vi "BME_Set_G05.vi"(0 "BME_G05P1 Settings":T2={"GateAB?"=FALSE, "Signal Type"=1, "InputTerminated?"=TRUE, "ClockEnabled?"=TRUE, "InternalClockPeriode(µs)"=1000000.0, "TriggerLevel"=1.25, "PresetValue"=0, "DivideBy"=8, "Clock Source"=1, "Gate Divider"=1, "PositiveGate?"=FALSE, "InternalTrigger?"=FALSE, "InternalArm?"=FALSE, "SWTrigger?"=FALSE, "RisingEdge?"=TRUE, "StopOnPreset?"=FALSE, "ResetWhenDone?"=FALSE, "TriggerEnabled?"=TRUE} {"Gate Divider" min=1 max=1000000; "Clock Source" items=["Internal Oscillator"=1, "External Trigger"=2, "Trigger & Oscillator"=3]; "Signal Type" items=["TTL"=1, "ECL"=2, "NIM"=3]}, 1 "DG_Number":i32, 5 "Chnl T":T1={" Delay (µs)"=0.0, "TriggerModulo"=1, "On? (false)"=FALSE, "PositiveVoltage?(true)"=TRUE, "50OhmTerminated? "=FALSE, "25OhmOutput?"=FALSE} {"TriggerModulo" min=1 max=1000000; "Delay (µs)" min=0.0 max=100000000.0 format="%.5f"}, 7 "Chnl A":T1={" Delay (µs)"=0.0, "TriggerModulo"=1, "On? (false)"=FALSE, "PositiveVoltage?(true)"=TRUE, "50OhmTerminated? "=FALSE, "25OhmOutput?"=FALSE} {"TriggerModulo" min=1 max=1000000; "Delay (µs)" min=0.0 max=100000000.0 format="%.5f"}, 9 "Chnl B":T1={" Delay (µs)"=0.0, "TriggerModulo"=1, "On? (false)"=FALSE, "PositiveVoltage?(true)"=TRUE, "50OhmTerminated? "=FALSE, "25OhmOutput?"=FALSE} {"TriggerModulo" min=1 max=1000000; "Delay (µs)" min=0.0 max=100000000.0 format="%.5f"}, 11 "error in (no error)":errorcluster) -> (8 "return value":i32, 15 "error out":errorcluster)   [LabVIEW 2009]
uses:
  BME_G05P1Settings.ctl
  SignalType.ctl
  ChnlWithModulo.ctl
  BME Beispiele/BME DLL/DelayGenerator.dll
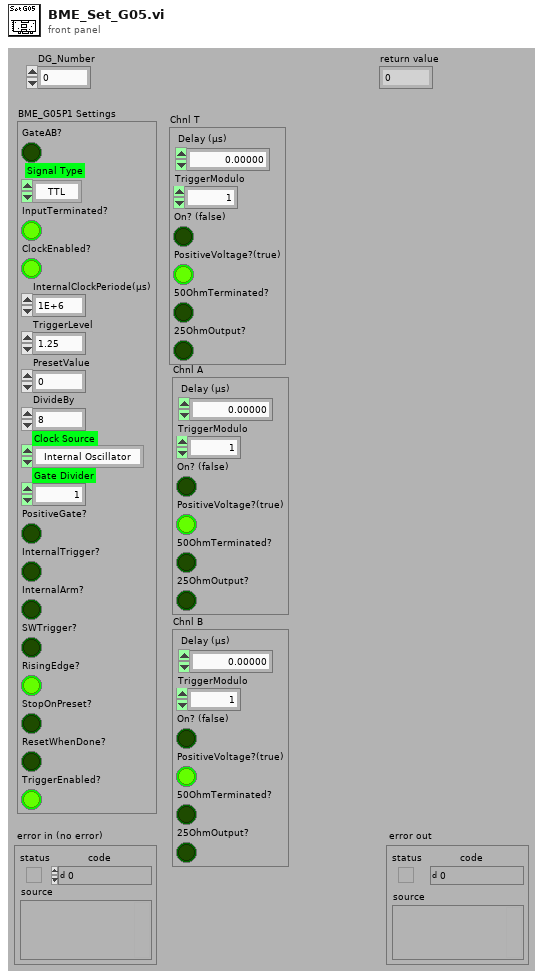
[diagram p1: front panel]
types:
  T1 = typedef "ChnlWithModulo.ctl" = cluster{" Delay (µs)":dbl, "TriggerModulo":u32, "On? (false)":bool, "PositiveVoltage?(true)":bool, "50OhmTerminated? ":bool, "25OhmOutput?":bool}
  T2 = typedef "BME_G05P1Settings.ctl" = cluster{"GateAB?":bool, "Signal Type":T3, "InputTerminated?":bool, "ClockEnabled?":bool, "InternalClockPeriode(µs)":dbl, "TriggerLevel":dbl, "PresetValue":i32, "DivideBy":i32, "Clock Source":u32, "Gate Divider":i32, "PositiveGate?":bool, "InternalTrigger?":bool, "InternalArm?":bool, "SWTrigger?":bool, "RisingEdge?":bool, "StopOnPreset?":bool, "ResetWhenDone?":bool, "TriggerEnabled?":bool}
  T3 = typedef "SignalType.ctl" = u32
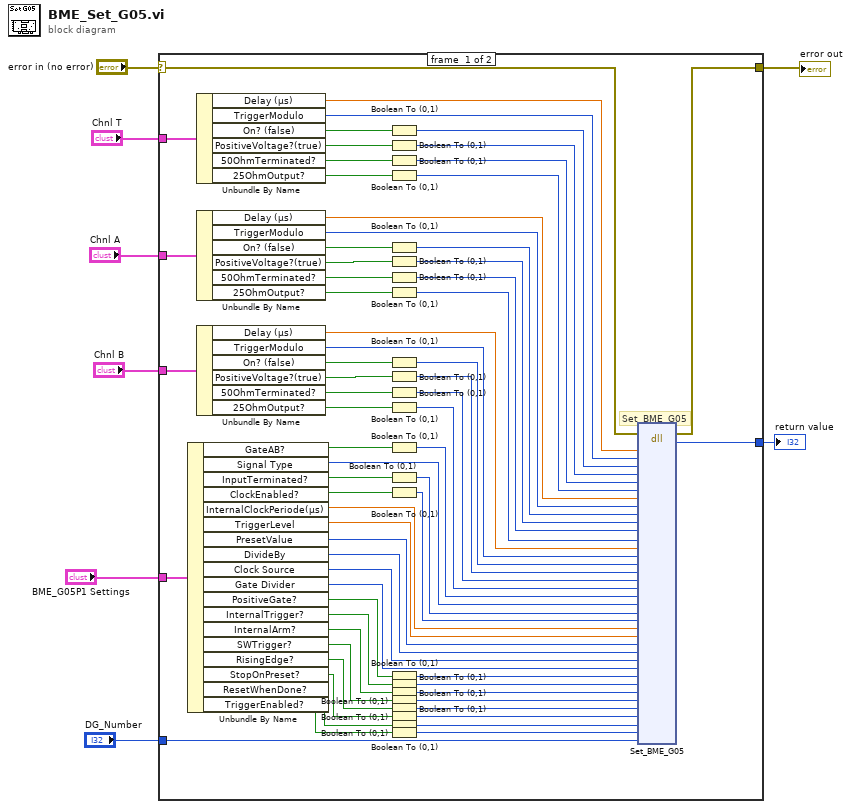
[diagram p0: block diagram]
diagram:
  n1 = case shown="No Error" "error in (no error)" {
    selector: "error in (no error)" -> [w9 w76]
    tunnel: "BME_G05P1 Settings" -> [w57 _]
    tunnel: "Chnl B" -> [w50 _]
    tunnel: "Chnl A" -> [w43 _]
    tunnel: "Chnl T" -> [w36 _]
    tunnel: [w34 _] -> w4
    tunnel: "DG_Number" -> [w33 _]
    tunnel: [w10 w76] -> w2
    frame #0 {
      # "Set_BME_G05"
      n2 = Unbundle By Name(w57) -> ("GateAB?"=w58:bool, "Signal Type"=w59:T3, "InputTerminated?"=w60:bool, "ClockEnabled?"=w61:bool, "InternalClockPeriode(µs)"=w62:dbl, "TriggerLevel"=w63:dbl, "PresetValue"=w64:i32, "DivideBy"=w65:i32, "Clock Source"=w66:u32, "Gate Divider"=w67:i32, "PositiveGate?"=w68:bool, "InternalTrigger?"=w69:bool, "InternalArm?"=w70:bool, "SWTrigger?"=w71:bool, "RisingEdge?"=w72:bool, "StopOnPreset?"=w73:bool, "ResetWhenDone?"=w74:bool, "TriggerEnabled?"=w75:bool)
      n3 = Unbundle By Name(w36) -> ("Delay (µs)"=w37:dbl, "TriggerModulo"=w38:u32, "On? (false)"=w39:bool, "PositiveVoltage?(true)"=w40:bool, "50OhmTerminated?"=w41:bool, "25OhmOutput?"=w42:bool)
      n4 = Unbundle By Name(w43) -> ("Delay (µs)"=w44:dbl, "TriggerModulo"=w45:u32, "On? (false)"=w46:bool, "PositiveVoltage?(true)"=w47:bool, "50OhmTerminated?"=w48:bool, "25OhmOutput?"=w49:bool)
      n5 = Unbundle By Name(w50) -> ("Delay (µs)"=w51:dbl, "TriggerModulo"=w52:u32, "On? (false)"=w53:bool, "PositiveVoltage?(true)"=w54:bool, "50OhmTerminated?"=w55:bool, "25OhmOutput?"=w56:bool)
      n6 = Boolean To (0,1)(Boolean=w39) -> (0, 1=w32:i16)
      n7 = Boolean To (0,1)(Boolean=w40) -> (0, 1=w31:i16)
      n8 = Boolean To (0,1)(Boolean=w41) -> (0, 1=w30:i16)
      n9 = Boolean To (0,1)(Boolean=w42) -> (0, 1=w29:i16)
      n10 = Boolean To (0,1)(Boolean=w46) -> (0, 1=w28:i16)
      n11 = Boolean To (0,1)(Boolean=w47) -> (0, 1=w27:i16)
      n12 = Boolean To (0,1)(Boolean=w48) -> (0, 1=w26:i16)
      n13 = Boolean To (0,1)(Boolean=w49) -> (0, 1=w25:i16)
      n14 = Boolean To (0,1)(Boolean=w53) -> (0, 1=w24:i16)
      n15 = Boolean To (0,1)(Boolean=w54) -> (0, 1=w23:i16)
      n16 = Boolean To (0,1)(Boolean=w55) -> (0, 1=w22:i16)
      n17 = Boolean To (0,1)(Boolean=w56) -> (0, 1=w21:i16)
      n18 = Boolean To (0,1)(Boolean=w58) -> (0, 1=w20:i16)
      n19 = Boolean To (0,1)(Boolean=w60) -> (0, 1=w19:i16)
      n20 = Boolean To (0,1)(Boolean=w61) -> (0, 1=w35:i16)
      n21 = Boolean To (0,1)(Boolean=w68) -> (0, 1=w18:i16)
      n22 = Boolean To (0,1)(Boolean=w69) -> (0, 1=w17:i16)
      n23 = Boolean To (0,1)(Boolean=w70) -> (0, 1=w16:i16)
      n24 = Boolean To (0,1)(Boolean=w71) -> (0, 1=w15:i16)
      n25 = Boolean To (0,1)(Boolean=w72) -> (0, 1=w14:i16)
      n26 = Boolean To (0,1)(Boolean=w73) -> (0, 1=w13:i16)
      n27 = Boolean To (0,1)(Boolean=w74) -> (0, 1=w12:i16)
      n28 = Boolean To (0,1)(Boolean=w75) -> (0, 1=w11:i16)
      n29 = dll-call lib="C:/Dokumente und Einstellungen/A2.5/Desktop/BME Beispiele/BME DLL/DelayGenerator.dll" fn="Set_BME_G05"(error in=w9, "T_0"=w37, "T0_output_modulo"=w38, "T0_active"=w32, "T0_pos"=w31, "T0_term"=w30, "T0_hdr"=w29, "T_a"=w44, "Ta_output_modulo"=w45, "A_active"=w28, "A_pos"=w27, "A_term"=w26, "A_hdr"=w25, "T_b"=w51, "Tb_output_modulo"=w52, "B_active"=w24, "B_pos"=w23, "B_term"=w22, "B_hdr"=w21, "Gate_AB"=w20, "Output Level"=w59, "Trg_term"=w19, "Clk_enable"=w35, "int_clock"=w62, "trg_level"=w63, "preset_val"=w64, "Divide_by"=w65, "Clock_Source"=w66, "Gate_Div"=w67, "gate_pos"=w18, "IntTrg"=w17, "IntArm"=w16, "software trg"=w15, "risingedge"=w14, "Stop_on_Preset"=w13, "ResetWhenDone"=w12, "TrgEnable"=w11, "DG_no"=w33) -> (error out=w10:errorcluster, "return type"=w34:i32)  [unwired: 39 in, 1 out]
    }
    frame #1 {
    }
  }
  "return value" <- w4
  "error out" <- w2
